vi "标样核查数据组合(子VI).vi"(9 "小时数据发送次数":i32, 10 "数据输入":string[][](array[string]), 11 "污染物编码":string) -> (3 "输出组合":string)   [LabVIEW 2016, in "数据传输系统-04.lvlib"]
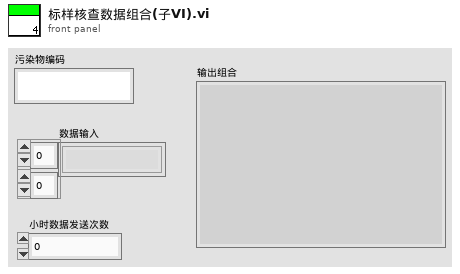
[diagram p1: front panel]
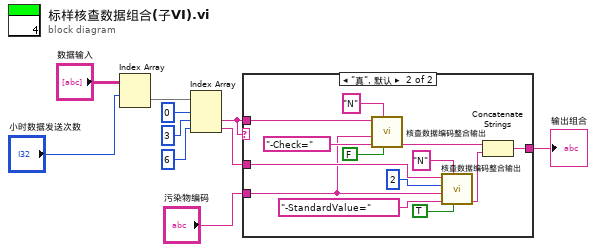
[diagram p0: block diagram]
diagram:
  n1 = Index Array(array="数据输入", index (row)="小时数据发送次数") -> (element=w8:string[])  [unwired: 1 in]
  n2 = Index Array(array=w8, index #1=0 ("索引"), index #2=3 ("索引"), index #3=6 ("索引")) -> (element #2=w4:string, element #3=w5:string)  [unwired: 1 out]
  n3 = case shown="\"真\", 默认" w4 {
    tunnel: w4 -> [w11 w23]
    tunnel: [w11 w20] -> w6
    tunnel: w5 -> [_ w16]
    tunnel: "污染物编码" -> [_ w12]
    frame "" {
    }
    frame "真", Default {
      n4 = call "核查数据编码整合输出.vi"("字段结束"=FALSE, "数据标识"="N" ("字符串"), "数据类型"="-Check=", "污染物编码"=w12, "数据值"=w23) -> ("编码输出"=w21:string)  [unwired: 6 in]
      n5 = call "核查数据编码整合输出.vi"("字段结束"=TRUE, "数据标识"="N" ("字符串"), "数据类型"="-StandardValue=", "污染物编码"=w12, "数据精度"=2, "数据值"=w16) -> ("编码输出"=w17:string)  [unwired: 5 in]
      n6 = Concatenate Strings(w21, w17) -> (w20:string)
    }
  }
  "输出组合" <- w6
